vi "SendToRecord.vi"(8 "error in (no error)":errorcluster) -> (0 "error out":errorcluster)   [LabVIEW 2015, in "MainController.lvlib"]
uses:
  MainController.lvlib
  <vilib>/addons/Qbus/Qbus.lvclass
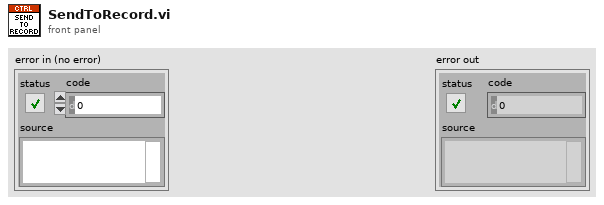
[diagram p1: front panel]
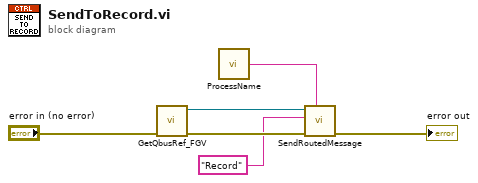
[diagram p0: block diagram]
diagram:
  n1 = call <vilib>:"GetQbusRef_FGV.vi"("error in (no error)"="error in (no error)") -> ("error out"=w5:errorcluster, "Qbus out"=w6:refnum<class "Qbus.lvclass">)  [unwired: 9 in]
  n2 = call "ProcessName.vi"() -> ("process name"=w4:string)  [unwired: 5 in]
  n3 = call <vilib>:"SendRoutedMessage.vi"("listener process"=w4, "error in (no error)"=w5, "message name"="Record", "Qbus in"=w6) -> ("error in (no error)"=→"error out":errorcluster)  [unwired: 6 in, 1 out]
